vi "LabJackT4_Main.vi"() -> ()   [LabVIEW 2019]
uses:
  sub/enum_dev_id.ctl
  <vilib>/Analysis/baseanly.llb/Mean (DBL).vi
  LabJackT4_Global.vi
  <vilib>/Analysis/NI_AALBase.lvlib
panel:
  out "HR3 Inlet":dbl format="%.4f"
  out "status":bool caption="Status"
  in  "logging_on":bool=TRUE
  out "log_st":bool
  out "TC_avg_degF":dbl format="%.1f"
  out "TC_avg_degC":dbl format="%.1f"
  out "array_ref_temp":dbl[](array[numeric]) caption="CJC" format="%_4g"
  out "Outside Tank":dbl format="%.1f"
  in  "Tab Control":T1(tab)
  out "chart_pres":waveform(dbl)[](graph)=[{"t0"=timestamp(3772890114.31303 s since 1904-01-01), "dt"=1.0, "Y"=[0.8687935985565186]}, {"t0"=timestamp(3772890114.31303 s since 1904-01-01), "dt"=1.0, "Y"=[86.87935985565186]}, {"t0"=timestamp(3772890114.31303 s since 1904-01-01), "dt"=1.0, "Y"=[30.48853325313992]}, {"t0"=timestamp(3772890114.31303 s since 1904-01-01), "dt"=1.0, "Y"=[303.6385332531399]}]
  in  "SPTD25":string="AIN0"
  in  "SPT25":string="AIN1"
  out "chart_pres_HR3":waveform(dbl)[](graph)=[{"t0"=timestamp(3772890114.31303 s since 1904-01-01), "dt"=1.0, "Y"=[0.8687935985565186]}, {"t0"=timestamp(3772890114.31303 s since 1904-01-01), "dt"=1.0, "Y"=[86.87935985565186]}, {"t0"=timestamp(3772890114.31303 s since 1904-01-01), "dt"=1.0, "Y"=[30.48853325313992]}, {"t0"=timestamp(3772890114.31303 s since 1904-01-01), "dt"=1.0, "Y"=[303.6385332531399]}]
  out "Chart degF":waveform(dbl)[](graph)
  out "Chart degC":waveform(dbl)[](graph)
  in  "LM34CAZ":string="AIN2"
  out "chart_ref_temp":waveform(dbl)[](graph)=[{"t0"=timestamp(3772890114.31303 s since 1904-01-01), "dt"=1.0, "Y"=[0.8687935985565186]}, {"t0"=timestamp(3772890114.31303 s since 1904-01-01), "dt"=1.0, "Y"=[86.87935985565186]}, {"t0"=timestamp(3772890114.31303 s since 1904-01-01), "dt"=1.0, "Y"=[30.48853325313992]}, {"t0"=timestamp(3772890114.31303 s since 1904-01-01), "dt"=1.0, "Y"=[303.6385332531399]}]
  out "chart_raw_v":waveform(dbl)[](graph)
  out "avg_data":dbl[](array[numeric])
  out "array_TC_degF":dbl[](array[numeric]) caption="TC degF" format="%_4g"
  out "array_TC_mV":dbl[](array[numeric]) caption="TC mV" format="%_4f"
  in  "amp_gain":dbl[](array[numeric])=[260.2, 260.0, 259.9, 259.8] format="%_4f"
  in  "amp_offset":dbl[](array[numeric])=[1.2648, 1.2687, 1.2357, 1.2546] format="%_5g"
  out "array_TC_degC":dbl[](array[numeric]) caption="TC degC" format="%_4g"
  in  "clear_chart":bool=TRUE caption="Clear charts to start"
  in  "dev_id":T2=enum."192.168.24.185"
  out "SN":i32
  in  "conn_type":T3(ring)=enum."LJM_ctETHERNET"
  out "Last Meas. Time":timestamp format="%<%Y-%m-%d %H:%M:%S>T"
  in  "Read Rate (Hz)":dbl=0.2 format="%#_15g"
  out "iter":i32 caption="Meas. count"
  in  "Scan Rate (Hz)":dbl=5000.0 format="%#.3f"
  in  "stop":bool
  out "Error Message":string
  # "Pressure & Temperature of Outside gHe Tank"
  # "LabJack T4"
  # "psi"
  # "psi"
  # "CH4"
  # "V"
  # "Bottom"
  # "degF"
  # "CH5"
  # "Right"
  # "CH6"
  # "Top"
  # "degC"
  # "CH7"
  # "K"
  # "Left"
  # "Average"
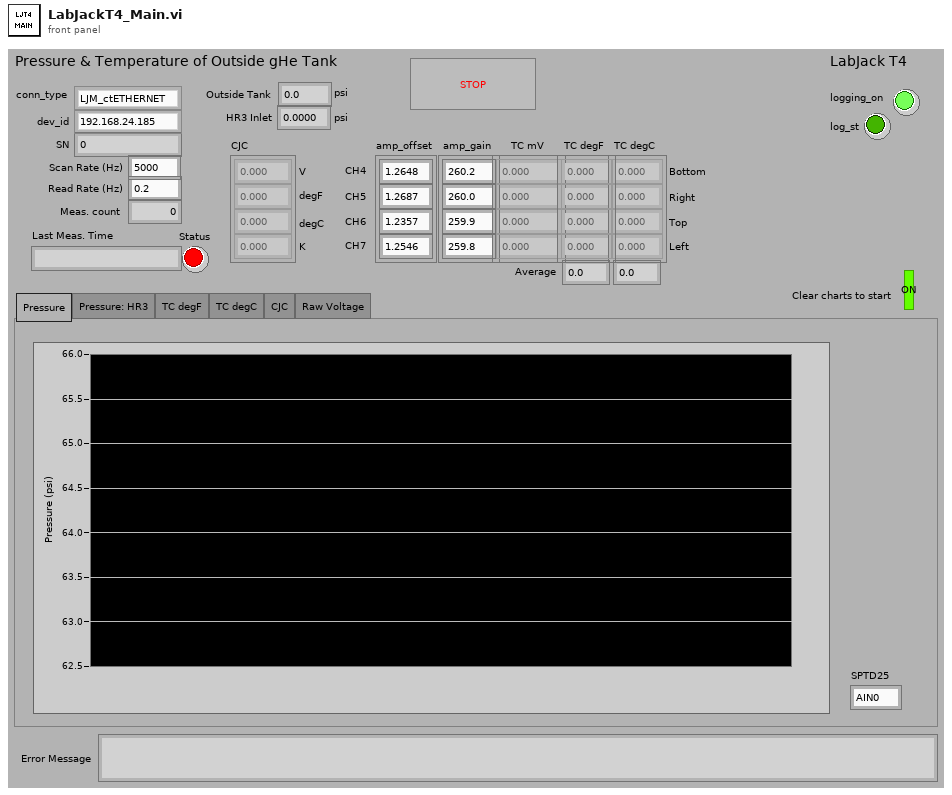
[diagram p1: front panel]
types:
  T1 = enum32{"Pressure", "Pressure: HR3", "TC degF", "TC degC", "CJC", "Raw Voltage"}
  T2 = typedef "enum_dev_id.ctl" = enum16{"LJM_idANY", "192.168.24.185", "10.0.0.176", "440017305"}
  T3 = enum16{"LJM_ctANY", "LJM_ctUSB", "LJM_ctETHERNET"}
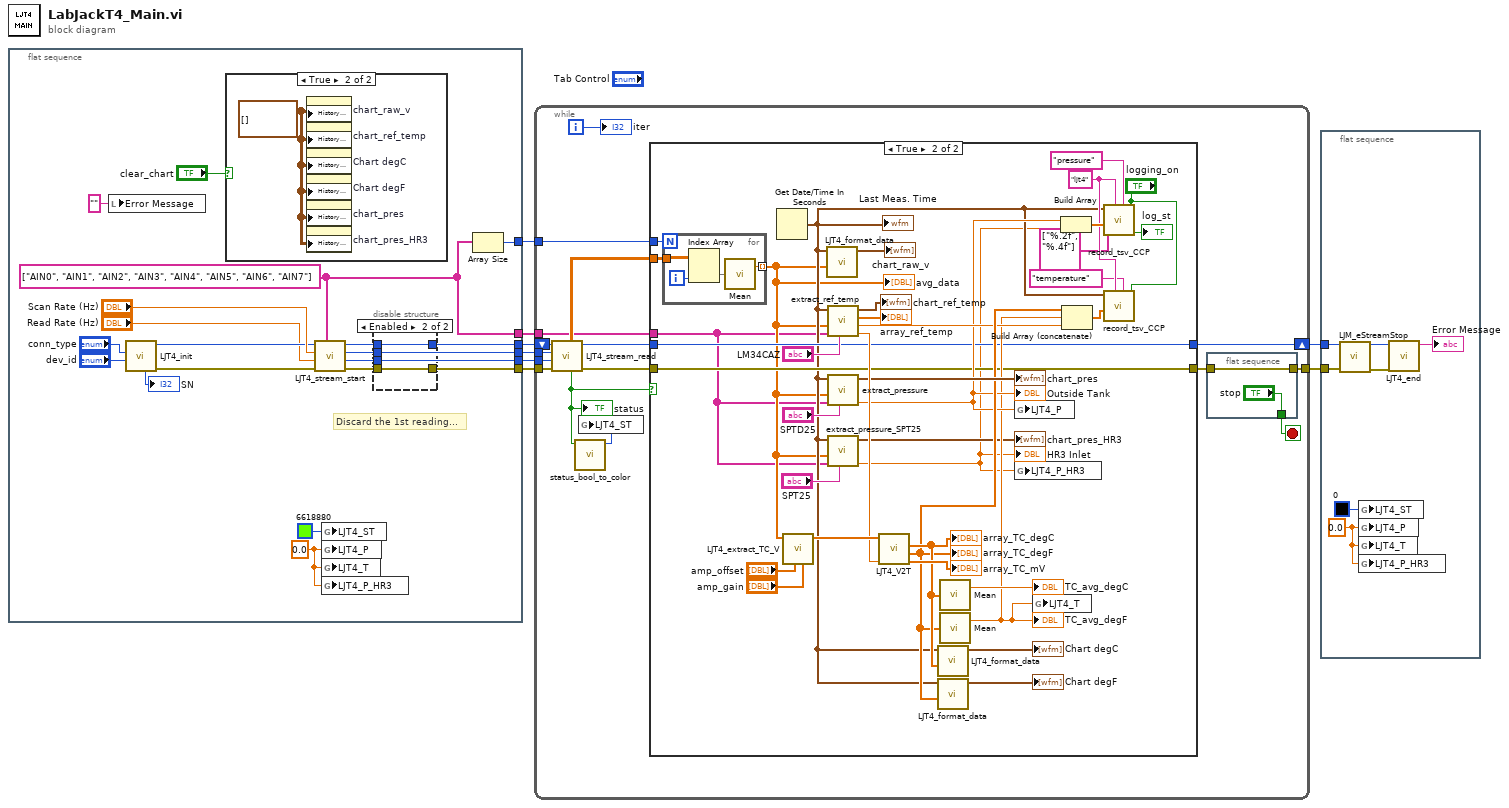
[diagram p0: block diagram]
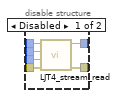
[diagram p2: hidden frame]
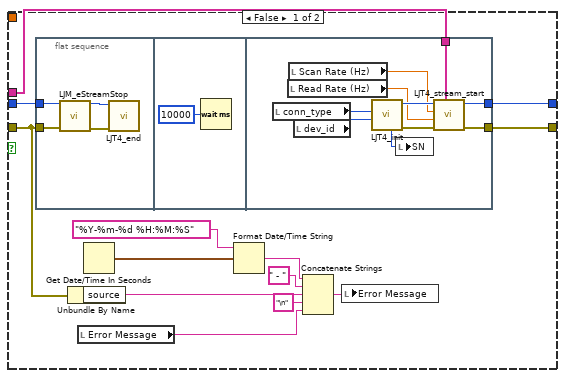
[diagram p4: hidden frame]
diagram:
  n1 = flat-sequence {
    tunnel: [w18] -> w8
    tunnel: [w17] -> w7
    tunnel: [w14] -> w4
    tunnel: [w15] -> w3
    tunnel: [w23] -> w2
    tunnel: [w12] -> w1
    frame #0 {
      w9 = 0.0 ("LJT4_P")
      w12 = string[] ["AIN0", "AIN1", "AIN2", "AIN3", "AIN4", "AIN5", "AIN6", "AIN7"] ("Scan List")
      # "Discard the 1st reading..."
      n2 = local write "Error Message"("" ("Error Message")) -> ()
      n3 = call "LJT4_init.vi"("dev_id"="dev_id", "conn_type"="conn_type") -> ("error out"=w26:errorcluster, "Handle Out"=w24:i32, "SN"=→"SN":i32)  [unwired: 5 in, 2 out]
      n4 = case shown="True" "clear_chart" {
        frame False {
        }
        frame True {
          w36 = waveform(dbl)[][] [] ("History Data")
          n5 = property on="chart_raw_v" class="WFChart (strict)"("History Data"=w36) -> ()  [unwired: 2 in, 2 out]
          n6 = property on="chart_ref_temp" class="WFChart (strict)"("History Data"=w36) -> ()  [unwired: 2 in, 2 out]
          n7 = property on="Chart degC" class="WFChart (strict)"("History Data"=w36) -> ()  [unwired: 2 in, 2 out]
          n8 = property on="Chart degF" class="WFChart (strict)"("History Data"=w36) -> ()  [unwired: 2 in, 2 out]
          n9 = property on="chart_pres" class="WFChart (strict)"("History Data"=w36) -> ()  [unwired: 2 in, 2 out]
          n10 = property on="chart_pres_HR3" class="WFChart (strict)"("History Data"=w36) -> ()  [unwired: 2 in, 2 out]
        }
      }
      n11 = call "LJT4_stream_start.vi"("Scan List"=w12, "error in"=w26, "Read Rate (Hz)"="Read Rate (Hz)", "Scan Rate (Hz)"="Scan Rate (Hz)", "Handle in"=w24) -> ("error out"=w27:errorcluster, "NumReadAddresses"=w14:i32, "ScansPerRead Out"=w15:i32, "Handle out"=w16:i32)  [unwired: 1 in, 2 out]
      n12 = global write "LabJackT4_Global.vi" "LJT4_ST"(u32 6618880 ("LJT4_ST")) -> ()
      n13 = global write "LabJackT4_Global.vi" "LJT4_P"(w9) -> ()
      n14 = global write "LabJackT4_Global.vi" "LJT4_T"(w9) -> ()
      n15 = global write "LabJackT4_Global.vi" "LJT4_P_HR3"(w9) -> ()
      n16 = disable-structure shown="Enabled" {
        disable-tunnel: w27 -> [w33 w34]
        disable-tunnel: [w32 w34] -> w18
        disable-tunnel: [w31 w35] -> w17
        disable-tunnel: w16 -> [w30 w35]
        disable-tunnel: w15 -> [w29 _]
        disable-tunnel: w14 -> [w28 _]
        frame Disabled {
          n17 = call "LJT4_stream_read.vi"("error in"=w33, "NumReadAddresses"=w28, "ScansPerRead"=w29, "Handle in"=w30) -> ("error out"=w32:errorcluster, "Handle Out"=w31:i32)  [unwired: 4 in, 2 out]
        }
        frame Enabled {
        }
      }
      n18 = Array Size(array=w12) -> (size(s)=w23:i32)
    }
  }
  n19 = while {
    tunnel: w4 -> [w49]
    tunnel: w3 -> [w48]
    tunnel: w8 -> [w51]
    tunnel: [w38] -> w6
    tunnel: w2 -> [w46]
    tunnel: w1 -> [w45]
    shift-right: [w40] -> w5
    shift-left: w7 -> [w50]
    i -> [w52]
    stop <- w37 stop-if-true
    n20 = call "LJT4_stream_read.vi"("error in"=w51, "NumReadAddresses"=w49, "ScansPerRead"=w48, "Handle in"=w50) -> ("error out"=w42:errorcluster, "Handle Out"=w41:i32, "status"=w43:bool, "data_out"=w47:dbl[][])  [unwired: 4 in]
    "status" <- w43
    n21 = call "status_bool_to_color.vi"("status_bool_1"=w43) -> ("status_color"=w44:u32)  [unwired: 10 in]
    n22 = global write "LabJackT4_Global.vi" "LJT4_ST"(w44) -> ()
    n23 = case shown="True" w43 {
      tunnel: w47 -> [_ w119]
      tunnel: w46 -> [_ w118]
      tunnel: w45 -> [w64 w85]
      tunnel: w42 -> [w63 w91]
      tunnel: [w66 w91] -> w39
      tunnel: w41 -> [w65 w90]
      tunnel: [w67 w90] -> w40
      frame False {
        n24 = flat-sequence {
          tunnel: w65 -> [w69]
          tunnel: w63 -> [w68]
          tunnel: [w77] -> w67
          tunnel: [w76] -> w66
          tunnel: w64 -> [w73]
          frame #0 {
            n25 = call "LJM_eStreamStop.vi"("Handle In"=w69, "error in"=w68) -> ("Handle Out"=w70:i32, "error out"=w71:errorcluster)  [unwired: 12 in]
            n26 = call "LJT4_end.vi"("error in"=w71, "Handle Out"=w70) -> ()  [unwired: 9 in, 1 out]
          }
          frame #1 {
            n27 = Wait (ms)(milliseconds to wait=u32 10000) -> ()  [unwired: 1 out]
          }
          frame #2 {
            n28 = local read "conn_type"() -> (w82:T3)
            n29 = local read "Read Rate (Hz)"() -> (w74:dbl)
            n30 = local read "Scan Rate (Hz)"() -> (w75:dbl)
            n31 = local read "dev_id"() -> (w81:T2)
            n32 = call "LJT4_init.vi"("dev_id"=w81, "conn_type"=w82) -> ("error out"=w79:errorcluster, "Handle Out"=w80:i32, "SN"=w78:i32)  [unwired: 5 in, 2 out]
            n33 = local write "SN"(w78) -> ()
            n34 = call "LJT4_stream_start.vi"("Scan List"=w73, "error in"=w79, "Read Rate (Hz)"=w74, "Scan Rate (Hz)"=w75, "Handle in"=w80) -> ("error out"=w76:errorcluster, "Handle out"=w77:i32)  [unwired: 1 in, 4 out]
          }
        }
        n35 = Unbundle By Name(w63) -> ("source"=w58:string)
        n36 = local read "Error Message"() -> (w56:string)
        n37 = Get Date/Time In Seconds() -> (seconds since 1Jan1904=w61:timestamp)
        n38 = Format Date/Time String(time format string (%c)="%Y-%m-%d %H:%M:%S", seconds (now)=w61) -> (date/time string=w60:string)  [unwired: 1 in]
        n39 = Concatenate Strings(w60, " - " ("string"), w58, "\n" ("string"), w56) -> (w55:string)
        n40 = local write "Error Message"(w55) -> ()
      }
      frame True {
        w100 = "ljt4" ("folder_name")
        n41 = for {
          N: w118 -> [_]
          tunnel: w119 -> [w123]
          tunnel: [w120] -> w86 mode=indexing
          i -> [w122]
          n42 = Index Array(array=w123, index (col)=w122) -> (element=w121:dbl[])  [unwired: 1 in]
          n43 = call-poly <vilib>:"Mean.vi"("X"=w121) -> ("mean"=w120:dbl)  [unwired: 1 out]
        }
        "avg_data" <- w86
        n44 = Get Date/Time In Seconds() -> (seconds since 1Jan1904=w87:timestamp)
        "Last Meas. Time" <- w87
        n45 = call "LJT4_extract_TC_V.vi"("amp_gain"="amp_gain", "amp_offset"="amp_offset", "voltage_raw"=w86) -> ("voltage_TC"=w113:dbl[])  [unwired: 7 in, 1 out]
        n46 = call "LJT4_format_data.vi"("value_array"=w86, "time"=w87) -> ("waveform_array_A"=→"chart_raw_v":waveform(dbl)[])  [unwired: 9 in]
        n47 = call "extract_ref_temp.vi"("name"="LM34CAZ", "name_array"=w85, "value_array"=w86, "time"=w87) -> ("temp_K"=w112:dbl, "temp_F"=w95:dbl, "temp_array"=→"array_ref_temp":dbl[], "waveform_array"=→"chart_ref_temp":waveform(dbl)[])  [unwired: 4 in]
        n48 = call "extract_pressure.vi"("name"="SPTD25", "name_array"=w85, "value_array"=w86, "time"=w87) -> ("P"=w93:dbl, "waveform_array"=→"chart_pres":waveform(dbl)[])  [unwired: 4 in, 2 out]
        "Outside Tank" <- w93
        n49 = call "extract_pressure_SPT25.vi"("name"="SPT25", "name_array"=w85, "value_array"=w86, "time"=w87) -> ("P"=w84:dbl, "waveform_array"=→"chart_pres_HR3":waveform(dbl)[])  [unwired: 5 in, 1 out]
        "HR3 Inlet" <- w84
        n50 = call "LJT4_V2T.vi"("CJC (K)"=w112, "voltage_array"=w113) -> ("array_mV"=→"array_TC_mV":dbl[], "array_T_F"=w96:dbl[], "array_T_C"=w104:dbl[])  [unwired: 6 in, 1 out]
        "array_TC_degC" <- w104
        "array_TC_degF" <- w96
        n51 = call "LJT4_format_data.vi"("value_array"=w104, "time"=w87) -> ("waveform_array_A"=→"Chart degC":waveform(dbl)[])  [unwired: 9 in]
        n52 = call "LJT4_format_data.vi"("value_array"=w96, "time"=w87) -> ("waveform_array_A"=→"Chart degF":waveform(dbl)[])  [unwired: 9 in]
        n53 = call-poly <vilib>:"Mean.vi"("X"=w104) -> ("mean"=→"TC_avg_degC":dbl)  [unwired: 1 out]
        n54 = call-poly <vilib>:"Mean.vi"("X"=w96) -> ("mean"=w92:dbl)  [unwired: 1 out]
        "TC_avg_degF" <- w92
        n55 = global write "LabJackT4_Global.vi" "LJT4_P"(w93) -> ()
        n56 = global write "LabJackT4_Global.vi" "LJT4_P_HR3"(w84) -> ()
        n57 = global write "LabJackT4_Global.vi" "LJT4_T"(w92) -> ()
        n58 = Build Array(w93, w84) -> (w101:dbl[])
        n59 = Build Array (concatenate)(w96, w92, w95) -> (w94:dbl[])
        n60 = call "record_tsv_CCP.vi"("logging_on"="logging_on", "file_name"="pressure", "folder_name"=w100, "format_array"=string[] ["%.2f", "%.4f"], "value_array"=w101, "time"=w87) -> ("status_log"=→"log_st":bool)  [unwired: 4 in, 1 out]
        n61 = call "record_tsv_CCP.vi"("logging_on"="logging_on", "file_name"="temperature", "folder_name"=w100, "value_array"=w94, "time"=w87) -> ()  [unwired: 5 in, 2 out]
      }
    }
    n62 = flat-sequence {
      tunnel: w39 -> [w54]
      tunnel: [w54] -> w38
      tunnel: ["stop"] -> w37
      frame #0 {
      }
    }
    "iter" <- w52
  }
  n63 = flat-sequence {
    tunnel: w6 -> [w130]
    tunnel: w5 -> [w129]
    frame #0 {
      w124 = 0.0 ("LJT4_P")
      n64 = call "LJM_eStreamStop.vi"("Handle In"=w129, "error in"=w130) -> ("Handle Out"=w127:i32, "error out"=w128:errorcluster)  [unwired: 12 in]
      n65 = global write "LabJackT4_Global.vi" "LJT4_ST"(u32 0 ("LJT4_ST")) -> ()
      n66 = global write "LabJackT4_Global.vi" "LJT4_P"(w124) -> ()
      n67 = global write "LabJackT4_Global.vi" "LJT4_T"(w124) -> ()
      n68 = global write "LabJackT4_Global.vi" "LJT4_P_HR3"(w124) -> ()
      n69 = call "LJT4_end.vi"("error in"=w128, "Handle Out"=w127) -> ("String"=→"Error Message":string)  [unwired: 9 in]
    }
  }
